vi "snap_action.vi"(0 "HGF_ImaqFg":refnum<class "HGF_ImaqFg.lvclass">, 2 "Image In":T1, 5 "error in (no error)":errorcluster, 6 "Region of Interest":i32[](array[numeric]), 7 "Step x":i32=-1, 8 "Channel":i32=-1, 9 "Step y":i32=-1) -> (14 "dup HGF_ImaqFg":refnum<class "HGF_ImaqFg.lvclass">, 16 "Image Out":T1, 19 "error out":errorcluster)   [LabVIEW 2014, in "HGF_IMAQ.lvlib" / "HGF_ImaqFg.lvclass"]
doc: "Acquires a single image into <B>Image out</B>. A snap is appropriate for low-speed or single-capture applications where ease of programming is essential."
uses:
  HGF_ImaqFg.lvclass
  <vilib>/vision/Image Controls.llb/IMAQ Image.ctl
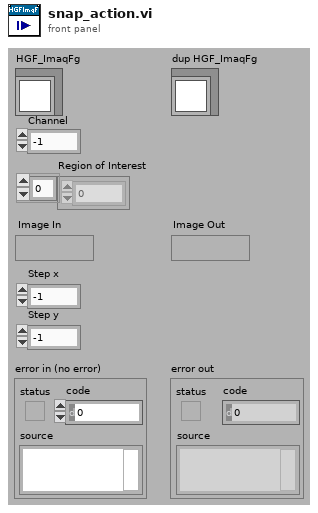
[diagram p1: front panel]
types:
  T1 = typedef "IMAQ Image.ctl" = refnum<image>
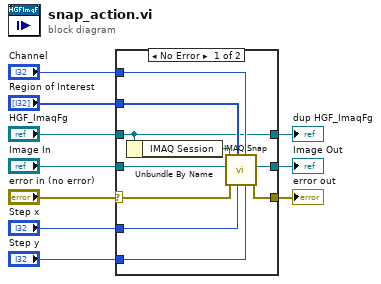
[diagram p0: block diagram]
diagram:
  n1 = case shown="No Error" "error in (no error)" {
    selector: "error in (no error)" -> [w19 w22]
    tunnel: "HGF_ImaqFg" -> [w12 w21]
    tunnel: "Image In" -> [w18 w23]
    tunnel: "Region of Interest" -> [w16 _]
    tunnel: "Step x" -> [w14 _]
    tunnel: "Channel" -> [w15 _]
    tunnel: "Step y" -> [w13 _]
    tunnel: [w17 w23] -> w4
    tunnel: [w12 w21] -> w3
    tunnel: [w11 w22] -> w1
    frame No Error {
      n2 = Unbundle By Name(w12) -> ("IMAQ Session"=w20:refnum<k11>)
      n3 = call <vilib>:"IMAQ Snap.vi"("Step y"=w13, "Channel"=w15, "Step x"=w14, "Region of Interest"=w16, "error in (no error)"=w19, "Image In"=w18, "IMAQ Session In"=w20) -> ("error out"=w11:errorcluster, "Image Out"=w17:T1)  [unwired: 3 out]
    }
    frame Error {
    }
  }
  "error out" <- w1
  "dup HGF_ImaqFg" <- w3
  "Image Out" <- w4
